vi "Scale Acquired Data.vi"(6 "range (V)":dbl=2.0, 9 "Sample Rate":dbl=800000000.0, 10 "Number of Bits":i16=12, 11 "Data In":u16[](array[numeric])=[51584, 51648, 51664, 51744, 51824, 51872, 51952, 52032, 52128, 52176, 52240, 52304, 52384, 52432, 52512, 52592, 52672, 52736, 52800, 52912, 52960, 53024, 53104, 53184, 53280, 53360, 53440, 53488, 53632, 53696, 53760, 53872, 53968, 54032, 54128, 54240, 54336, 54416, 54512, 54592, 54720, 54720, 54864, 54944, 55056, 55136, 55232, 55328, 55440, 55520, 55616, 55760, 55888, 55936, 56064, 56160, 56224, 56368, 56432, 56560, 56672, 56768, 56832, 56960, 57072, 57200, 57296, 57376, 57504, 57600, 57744, 57824, 57936, 58064, 58144, 58224, 58352, 58480, 58592, 58704, 58800, 58944, 59072, 59168, 59312, 59408, 59568, 59664, 59728, 59904, 60032, 60128, 60256, 60384, 60480, 60608, 60688, 60864, 60992, 61104, 61200, 61312, 61456, 61584, 61680, 61792, 61888, 62048, 62176, 62256, 62384, 62528, 62672, 62784, 62944, 63072, 63184, 63296, 63472, 63584, 63712, 63856, 63968, 64080, 64224, 64320, 64464, 64576, 64720, 64816, 64976, 65088, 65184, 65312, 65440, 16, 144, 272, 384, 480, 672, 768, 848, 1040, 1136, 1296, 1408, 1536, 1680, 1760, 1936, 2016, 2176, 2272, 2416, 2528, 2672, 2784, 2944, 3056, 3152, 3296, 3424, 3520, 3680, 3760, 3888, 4000, 4112, 4256, 4384, 4464, 4640, 4784, 4880, 4992, 5104, 5232, 5344, 5456, 5568, 5696, 5808, 5936, 6064, 6192, 6256, 6400, 6512, 6624, 6752, 6832, 6976, 7120, 7216, 7312, 7424, 7552, 7616, 7776, 7840, 7968, 8064, 8160, 8288, 8384, 8480, 8608, 8752, 8848, 8944, 9024, 9136, 9296, 9392, 9472, 9568, 9696, 9776, 9856, 9968, 10080, 10192, 10240, 10352, 10448, 10560, 10608, 10736, 10816, 10912, 10976, 11088, 11184, 11312, 11376, 11424, 11520, 11616, 11712, 11824, 11904, 11968, 12032, 12160, 12240, 12336, 12368, 12448, 12560, 12640, 12752, 12800, 12864, 12960, 12992, 13072, 13136, 13232, 13312, 13424, 13456, 13504, 13600, 13648, 13728, 13776, 13856, 13920, 13984, 14000, 14080, 14144, 14192, 14272, 14336, 14368, 14432, 14512, 14544, 14640, 14656, 14688, 14752, 14800, 14832, 14880, 14928, 14992, 15040, 15120, 15184, 15200, 15248, 15264, 15312, 15360, 15376, 15408, 15488, 15504, 15504, 15552, 15600, 15584, 15632, 15680, 15712, 15744, 15744, 15792, 15808, 15808, 15872, 15888, 15888, 15904, 15888, 15952, 15984, 15984, 16032, 16032, 16048, 16032, 16064, 16048, 16064, 16064, 16096, 16080, 16096, 16080, 16064, 16096, 16112, 16128, 16144, 16096, 16080, 16096, 16096, 16048, 16064, 16048, 16032, 16032, 16000, 15984, 16016, 15984, 15968, 15968, 15968, 15904, 15872, 15856, 15856, 15840, 15792, 15792, 15760, 15744, 15728, 15648, 15648, 15600, 15584, 15584, 15552, 15488, 15456, 15424, 15376, 15328, 15280, 15264, 15232, 15168, 15152, 15072, 15024, 15008, 14944, 14880, 14832, 14768, 14720, 14688, 14672, 14592, 14544, 14480, 14448, 14368, 14320, 14256, 14224, 14144, 14112, 14016, 13984, 13904, 13856, 13792, 13728, 13664, 13568, 13504, 13440, 13344, 13344, 13280, 13168, 13104, 13024, 12960, 12848, 12800, 12704, 12624, 12544, 12480, 12400, 12272, 12256, 12160, 12048, 11984, 11904, 11808, 11680, 11616, 11552, 11440, 11344, 11264, 11168, 11104, 11024, 10896, 10816, 10752, 10640, 10560, 10432, 10320, 10272, 10144, 10080, 9984, 9904, 9776, 9648, 9568, 9488, 9392, 9264, 9168, 9072, 8944, 8832, 8736, 8576, 8528, 8400, 8336, 8208, 8096, 7952, 7840, 7696, 7632, 7520, 7392, 7280, 7168, 7088, 6960, 6848, 6736, 6624, 6464, 6384, 6256, 6176, 6032, 5904, 5760, 5696, 5536, 5456, 5296, 5216, 5088, 4976, 4864, 4736, 4576, 4496, 4384, 4240, 4128, 3984, 3872, 3760, 3664, 3504, 3360, 3264, 3136, 3040, 2912, 2752, 2640, 2480, 2400, 2272, 2128, 2016, 1856, 1808, 1600, 1504, 1376, 1264, 1120, 1008, 832, 752, 640, 480, 352, 240, 128, 16, 65408, 65296, 65216, 65056, 64928, 64784, 64656, 64544, 64448, 64320, 64144, 64032, 63920, 63744, 63648, 63520, 63376, 63296, 63168, 63024, 62880, 62752, 62624, 62512, 62352, 62256, 62176, 61984, 61888, 61744, 61616, 61520, 61392, 61232, 61152, 61072, 60912, 60800, 60672, 60560, 60432, 60272, 60176, 60064, 60000, 59840, 59696, 59600, 59488, 59376, 59248, 59104, 59008, 58896, 58752, 58672, 58528, 58448, 58336, 58224, 58112, 58048, 57920, 57760, 57664, 57568, 57472, 57328, 57216, 57168, 57040, 56944, 56784, 56736, 56592, 56512, 56368, 56288, 56192, 56112, 56000, 55904, 55776, 55696, 55568, 55472, 55376, 55296, 55216, 55120, 54992, 54912, 54784, 54784, 54640, 54560, 54464, 54384, 54272, 54192, 54096, 54000, 53904, 53808, 53712, 53664, 53568, 53440, 53408, 53312, 53248, 53168, 53104, 53008, 52944, 52864, 52768, 52672, 52608, 52528, 52480, 52384, 52352, 52256, 52208, 52128, 52080, 52000, 51920, 51888, 51808, 51712, 51664, 51600, 51552, 51472, 51440, 51376, 51296, 51264, 51184, 51168, 51088, 51056, 50960, 50944, 50864, 50816, 50768, 50704, 50640, 50640, 50592, 50512, 50480, 50448, 50368, 50336, 50304, 50272, 50272, 50224, 50192, 50144, 50096, 50064, 50000, 50016, 49984, 49920, 49872, 49872, 49840, 49824, 49808, 49792, 49792, 49760, 49728, 49680, 49712, 49664, 49648, 49680, 49648, 49632, 49648, 49616, 49584, 49568, 49552, 49568, 49552, 49552, 49536, 49504, 49536, 49536, 49520, 49536, 49568, 49536, 49520, 49536, 49536, 49520, 49552, 49536, 49584, 49584, 49584, 49616, 49616, 49648, 49648, 49648, 49664, 49696, 49712, 49744, 49728, 49744, 49792, 49792, 49792, 49840, 49904, 49888, 49936, 49984, 50016, 50064, 50048, 50112, 50128, 50128, 50176, 50240, 50272, 50288, 50320, 50400, 50416, 50464, 50496, 50560, 50608, 50640, 50688, 50768, 50816, 50864, 50896, 50928, 50992, 51056, 51104, 51184, 51232, 51280, 51376, 51424, 51440, 51536, 51568, 51648, 51696, 51776, 51856, 51920, 51968, 52048, 52096, 52192, 52256, 52336, 52400, 52448, 52544, 52560, 52672, 52752, 52832, 52944, 52976, 53040, 53152, 53184, 53264, 53312, 53424, 53568, 53632, 53680, 53776, 53840, 53952, 54064, 54160, 54240, 54304, 54400, 54512, 54592, 54704, 54816, 54896, 54976, 55040, 55200, 55248, 55360, 55456, 55552, 55648, 55728, 55824, 55936, 56032, 56160, 56224, 56304, 56432, 56512, 56640, 56752, 56912, 56960, 57040, 57184, 57280, 57392, 57536, 57616, 57760, 57840, 57952, 58064, 58128, 58240, 58368, 58512, 58592, 58720, 58864, 58960, 59056, 59184, 59328, 59424, 59552, 59680, 59808, 59920, 60032, 60176, 60272, 60384, 60496, 60624, 60688, 60832, 60960, 61072, 61200, 61328, 61440, 61568, 61680, 61840, 61936, 62128, 62208, 62320, 62400, 62544, 62672, 62816, 62912, 63056, 63184, 63344, 63440, 63584, 63696, 63840, 63952, 64048, 64224, 64336, 64480, 64592, 64704, 64816, 64928, 65104, 65216, 65328, 65456, 80, 128, 272, 384, 512, 656, 752, 896, 1040, 1152, 1264, 1424, 1520, 1680, 1792, 1904, 2016, 2160, 2288, 2432, 2528, 2672, 2816, 2928, 3040, 3184, 3280, 3424, 3568, 3664, 3776, 3920, 4000, 4160, 4256, 4416, 4544, 4624, 4768, 4848, 4960, 5120, 5232, 5312, 5440, 5568, 5696, 5792, 5952, 6048, 6176, 6256, 6416, 6512, 6624, 6736, 6880, 7024, 7104, 7200, 7344, 7392, 7536, 7632, 7776, 7888, 8000, 8080, 8176, 8304, 8368, 8496, 8624, 8720, 8848, 8960, 9056, 9168, 9280, 9392, 9488, 9584, 9696, 9824, 9872, 10016, 10064, 10160, 10288, 10352, 10448, 10576, 10656, 10736, 10848, 10944, 11040, 11088, 11216, 11296, 11376, 11472, 11568, 11632, 11728, 11808, 11904, 11968, 12048, 12128, 12240, 12320, 12400, 12512, 12576, 12624, 12720, 12800, 12896, 12928, 13008, 13120, 13152, 13264, 13344, 13376, 13424, 13520, 13584, 13680, 13712, 13776, 13872, 13936, 13984, 14064, 14096, 14144, 14224, 14288, 14336, 14368, 14432, 14464, 14544, 14608, 14656, 14720, 14752, 14800, 14832, 14864, 14944, 15008, 15088, 15120, 15136, 15200, 15232, 15264, 15296, 15360, 15392, 15424, 15488, 15504, 15536, 15584, 15616, 15664, 15664, 15680, 15712, 15760, 15808, 15792, 15824, 15840, 15856, 15872, 15904, 15936, 15968, 15936, 16000, 15952, 16032, 16016, 16048, 16048, 16048, 16080, 16064, 16080, 16112, 16128, 16128, 16080, 16080, 16096, 16096, 16080, 16080, 16064, 16096, 16080, 16112, 16064, 16048, 16048, 16048, 16032, 16032, 16000, 15968, 15984, 15968, 15984, 15952, 15920, 15888, 15888, 15888, 15856, 15824, 15808, 15760, 15744, 15680, 15664, 15648, 15632, 15632, 15584, 15520, 15504, 15472, 15408, 15376, 15328, 15312, 15312, 15216, 15216, 15152, 15104, 15072, 15024, 14960, 14864, 14864, 14800, 14752, 14688, 14672, 14544, 14544, 14464, 14448, 14368, 14320, 14272, 14224, 14144, 14128, 14064, 13984, 13920, 13872, 13792, 13728, 13680, 13584, 13504, 13440, 13392, 13312, 13280, 13200, 13104, 13056, 12944, 12864, 12784, 12720, 12640, 12544, 12464, 12368, 12352, 12256, 12144, 12032, 11968, 11904, 11824, 11744, 11632, 11552, 11456, 11392, 11312, 11216, 11136, 11008, 10896, 10848, 10736, 10640, 10544, 10464, 10384, 10240, 10176, 10080, 10000, 9888, 9808, 9680, 9552, 9472, 9376, 9280, 9168, 9088, 8976, 8816, 8752, 8624, 8496, 8416, 8320, 8192, 8080, 7984, 7872, 7728, 7680, 7504, 7424, 7296, 7184, 7056, 6976, 6832, 6720, 6624, 6528, 6416, 6288, 6160, 6032, 5920, 5808, 5680, 5552, 5456, 5328, 5200, 5072, 4928, 4864, 4720, 4592, 4464, 4336, 4240, 4128, 4016, 3888, 3760, 3648, 3536, 3392, 3248, 3136, 3008, 2912, 2800, 2704, 2560, 2384, 2256, 2096, 2032, 1888, 1776, 1616, 1504, 1408, 1248, 1104, 1008, 848, 752, 592, 480, 352, 240, 128, 0, 65408, 65280, 65184, 65040, 64912, 64800, 64688, 64528, 64416, 64304, 64176, 64064, 63936, 63744, 63632, 63520, 63392, 63280, 63136, 63024, 62896, 62768, 62624, 62464, 62368, 62240, 62144, 62016, 61856, 61776, 61632, 61504, 61360, 61280, 61152, 61024, 60928, 60832, 60688, 60560, 60416, 60288, 60208, 60064, 59952, 59824, 59712, 59584, 59472, 59312, 59280, 59152, 58992, 58944, 58784, 58704, 58544, 58448, 58336, 58208, 58128, 58016, 57888, 57824, 57712, 57568, 57472, 57344, 57264, 57136, 57008, 56912, 56800, 56720, 56624, 56512, 56416, 56304, 56192, 56096, 55984, 55936, 55792, 55696, 55600, 55488, 55408, 55312, 55184, 55088, 55024, 54896, 54848, 54736, 54688, 54576, 54464, 54384, 54288, 54160, 54096, 54016, 53904, 53824, 53712, 53648, 53568, 53472, 53360, 53296, 53248, 53184, 53088, 53008, 52912, 52864, 52768, 52720, 52640, 52544, 52496, 52400, 52320, 52256, 52192, 52128, 52064, 52016, 51952, 51888, 51776, 51728, 51664, 51632, 51552, 51488, 51392, 51360, 51312, 51248, 51168, 51136, 51072, 51008, 50944, 50928, 50848, 50768, 50736, 50704, 50672, 50592, 50560, 50512, 50480, 50448, 50384, 50352, 50304, 50256, 50256, 50208, 50144, 50128, 50080, 50080, 50016, 50032, 49984, 49952, 49920, 49856, 49856, 49840, 49824, 49792, 49760, 49728, 49712, 49712, 49712, 49696, 49680, 49680, 49632, 49632, 49568, 49648, 49584, 49584, 49552, 49568, 49552, 49552, 49520, 49552, 49536, 49520, 49536, 49520, 49504, 49520, 49552, 49568, 49552, 49584, 49584, 49568, 49584, 49568, 49632, 49648, 49648, 49664, 49664, 49648, 49680, 49696, 49728, 49712, 49776, 49792, 49792, 49840, 49840, 49888, 49904, 49888, 49904, 49952, 50016, 50032, 50080, 50112, 50128, 50144, 50208, 50256, 50272, 50304, 50368, 50400, 50432, 50480, 50528, 50560, 50592, 50672, 50688, 50768, 50784, 50832, 50896, 50944, 51008, 51072, 51136, 51184, 51216, 51312, 51360, 51424, 51456, 51536, 51648, 51664, 51712, 51776, 51856, 51904, 52016, 52064, 52112, 52192, 52224, 52368, 52368, 52448, 52544, 52592, 52656, 52768, 52848, 52912, 52992, 53024, 53136, 53200, 53280, 53392, 53488, 53536, 53632, 53696, 53792, 53920, 53952, 54080, 54128, 54240, 54320, 54400, 54496, 54624, 54704, 54784, 54880, 54976, 55072, 55168, 55264, 55344, 55456, 55552, 55664, 55728, 55856, 55936, 56032, 56176, 56256, 56368, 56432, 56560, 56672, 56800, 56880, 57024, 57072, 57152, 57280, 57392, 57536, 57632, 57728, 57856, 57968, 58048, 58144, 58272, 58384, 58480, 58608, 58720, 58816, 58944, 59072, 59200, 59328, 59456, 59536, 59648, 59776, 59936, 60048, 60128, 60240, 60384, 60512, 60624, 60736, 60848, 61008, 61088, 61216, 61328, 61456, 61616, 61696, 61824, 61920, 62032, 62208, 62320, 62448, 62576, 62704, 62816, 62944, 63088, 63184, 63312, 63440, 63536, 63680, 63856, 63952, 64064, 64192, 64320, 64432, 64576, 64704, 64864, 64960, 65072, 65216, 65312, 65424, 32, 144, 288, 416, 512, 640, 752, 912, 1056, 1184, 1296, 1440, 1536, 1648, 1792, 1952, 2016, 2176, 2336, 2432, 2560, 2704, 2784, 2960, 3040, 3136, 3312, 3440, 3552, 3616, 3744, 3920, 4000, 4144, 4240, 4400, 4528, 4656, 4752, 4864, 4960, 5104, 5232, 5360, 5472, 5584, 5696, 5824, 5936, 6032, 6176, 6256, 6416, 6544, 6640, 6752, 6864, 6976, 7088, 7184, 7296, 7392, 7520, 7632, 7776, 7888, 7952, 8096, 8208, 8272, 8384, 8512, 8624, 8736, 8832, 8976, 9088, 9200, 9280, 9424, 9504, 9568, 9696, 9808, 9888, 9984, 10096, 10176, 10256, 10352, 10464, 10544, 10640, 10720, 10832, 10896, 10992, 11104, 11184, 11296, 11392, 11440, 11536, 11632, 11696, 11824, 11888, 11984, 12064, 12160, 12240, 12336, 12400, 12496, 12544, 12608, 12704, 12816, 12864, 12960, 13024, 13104, 13168, 13248, 13344, 13376, 13472, 13520, 13584, 13664, 13728, 13808, 13904, 13936, 14016, 14048, 14080, 14176, 14208, 14288, 14320, 14368, 14416, 14544, 14544, 14624, 14672, 14736, 14752, 14800, 14896, 14928, 14960, 15024, 15072, 15152, 15216, 15248, 15264, 15312, 15344, 15376, 15392, 15440, 15456, 15504, 15584, 15584, 15616, 15680, 15648, 15664, 15712, 15728, 15792, 15808, 15792, 15856, 15856, 15888, 15936, 15936, 15920, 15936, 15968, 16000, 16016, 16016, 16032, 16032, 16048, 16080, 16064, 16080, 16080, 16128, 16144, 16112, 16128, 16096, 16112, 16096, 16096, 16064, 16096, 16080, 16080, 16096, 16080, 16080, 16080, 16032, 16032, 16016, 16032, 15968, 15984, 15984, 15936, 15936, 15920, 15904, 15856, 15824, 15808, 15808, 15792, 15776, 15744, 15696, 15696, 15648, 15616, 15616, 15536, 15504, 15472, 15408, 15360, 15344, 15280, 15248, 15232, 15216, 15104, 15104, 15024, 14976, 14960, 14896, 14832, 14800, 14736, 14688, 14624, 14576, 14544, 14496, 14432, 14368, 14352, 14256, 14208, 14176, 14096, 14048, 13984, 13920, 13856, 13824, 13760, 13664, 13600, 13488, 13472, 13392, 13360, 13248, 13216, 13104, 13040, 12912, 12864, 12800, 12720, 12640, 12528, 12464, 12400, 12336, 12304, 12176, 12032, 11968, 11904, 11808, 11760, 11648, 11536, 11472, 11392, 11296, 11200, 11104, 11040, 10912, 10800, 10752, 10656, 10576, 10432, 10336, 10256]) -> (3 "output waveform":waveform(ext))   [LabVIEW 2017]
doc: "This VI scales the raw data returned by the adapter module from ADC codes to volts. It also stores the data in a waveform data type and sets the sample rate for the waveform."
panel:
  # "Refer to the Block Diagram of this VI for execution comments."
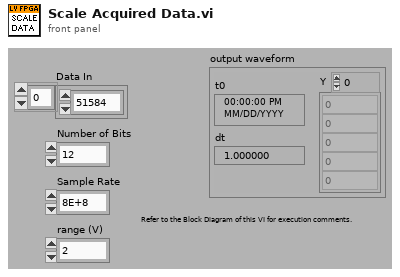
[diagram p1: front panel]
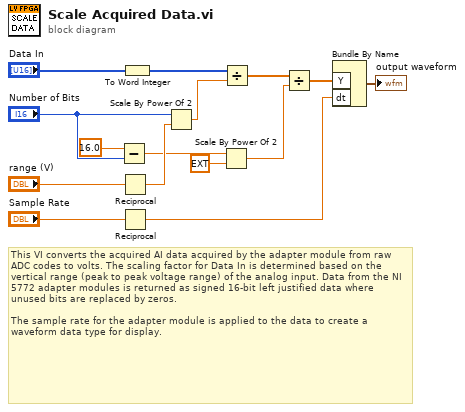
[diagram p0: block diagram]
diagram:
  # "This VI converts the acquired AI data acquired by the adapter module from raw ADC codes to volts. The scaling factor for Data In is determined based on the vertical range (peak to peak voltage range) of the analog input. Data from the NI 5772 adapter modules is returned as signed 16-bit left justified data where unused bits are replaced by zeros.  \n\nThe sample rate for the adapter module is applied to the data to create a waveform data type for display."
  n1 = Subtract(x=16.0 ("y"), y="Number of Bits") -> (x-y=w4:dbl)
  n2 = Reciprocal(x="range (V)") -> (1/x=w13:dbl)
  n3 = Reciprocal(x="Sample Rate") -> (1/x=w15:dbl)
  n4 = To Word Integer(number="Data In") -> (16bit integer=w8:i16[])
  n5 = Scale By Power Of 2(n="Number of Bits", x=w13) -> (x*2^n=w14:dbl)
  n6 = Scale By Power Of 2(n=w4, x=ext 1.0) -> (x*2^n=w2:ext)
  n7 = Divide(x=w8, y=w14) -> (x/y=w9:dbl[])
  n8 = Divide(x=w9, y=w2) -> (x/y=w7:ext[])
  n9 = Bundle By Name("Y"=w7, "dt"=w15) -> (→"output waveform":waveform(ext))  [unwired: 1 out]
